vi "Write LEDs.vi"(8 "error in (no error)":errorcluster, 10 "LED Engine Refs in":T1 {"RT IDs"."Slot #" max=15; "RT IDs"."Chip Address (A2 A1 A0)" max=7; "RT Block Data Refs"."Data Reference" format="%.0x"}, 11 "DMA FIFO Ref in":refnum<k20>) -> (0 "error out":errorcluster, 2 "LED Engine Refs out":T1 {"RT IDs"."Slot #" max=15; "RT IDs"."Chip Address (A2 A1 A0)" max=7; "RT Block Data Refs"."Data Reference" format="%.0x"})   [LabVIEW 2014, in "SLSC configuration Engine.lvlib"]
uses:
  SLSC configuration Engine.lvlib
  Type Defs/RT Engine Refs.ctl
  Shared/Type Defs/RT IDs.ctl
  Shared/SPI Utility/Slot #.ctl
  Shared/MCP23S17/Chip Address.ctl
  <vilib>/NI Veristand/Custom Device API/Block Data Reference.ctl
  <vilib>/NI Veristand/Custom Device API/Data Reference.ctl
  <vilib>/NI Veristand/Custom Device API/Global Data Refs.vi
  Shared/Constants.vi
  <vilib>/NI Veristand/Custom Device API/Custom Device API.lvlib
  Shared/SLSC configuration Shared.lvlib
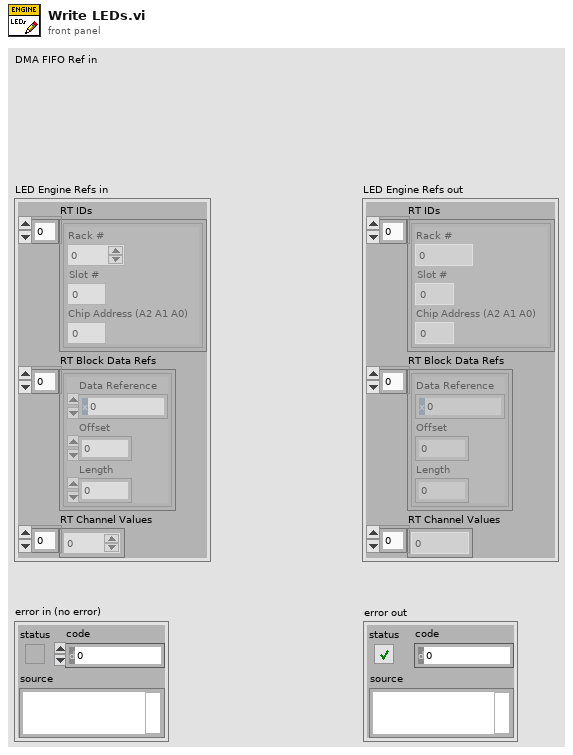
[diagram p1: front panel]
types:
  T1 = typedef "SLSC configuration Engine.lvlib/RT Engine Refs.ctl" = cluster{"RT IDs":T2[], "RT Block Data Refs":T5[], "RT Channel Values":dbl[]}
  T2 = typedef "SLSC configuration Shared.lvlib/RT IDs.ctl" = cluster{"Rack #":u8, "Slot #":T3, "Chip Address (A2 A1 A0)":T4}
  T3 = typedef "SLSC configuration Shared.lvlib/Slot #.ctl" = u8
  T4 = typedef "SLSC configuration Shared.lvlib/Chip Address.ctl" = u8
  T5 = typedef "Custom Device API.lvlib/Block Data Reference.ctl" = cluster{"Data Reference":T6, "Offset":i32, "Length":i32}
  T6 = typedef "Custom Device API.lvlib/Data Reference.ctl" = i32
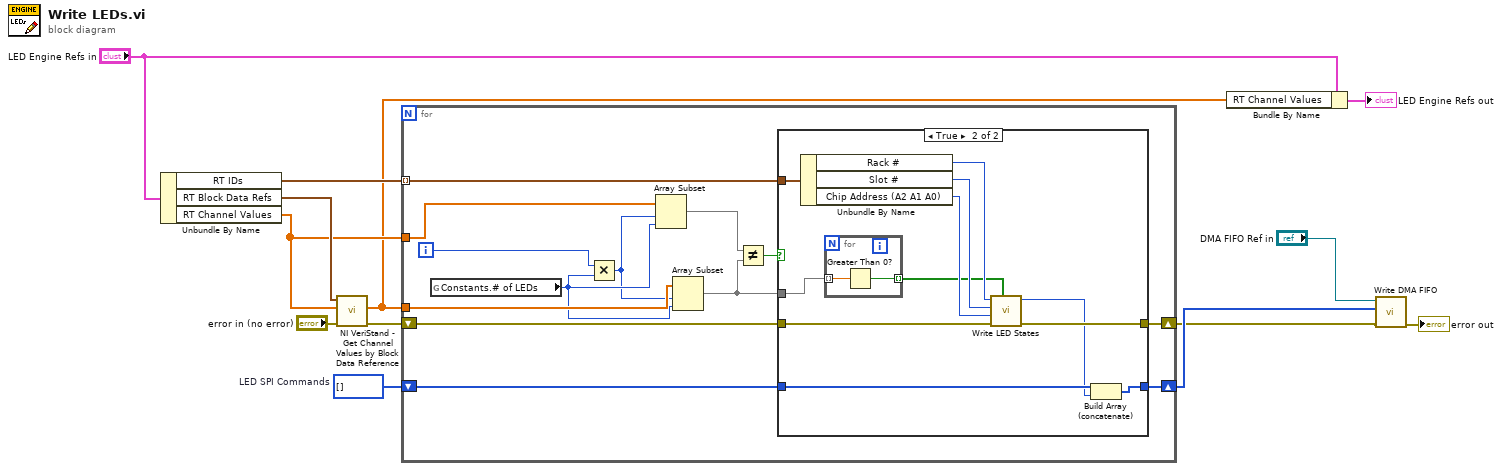
[diagram p0: block diagram]
diagram:
  w5 = u64[] []  # LED SPI Commands
  n1 = Unbundle By Name("LED Engine Refs in") -> ("RT IDs"=w10:T2[], "RT Block Data Refs"=w13:T5[], "RT Channel Values"=w8:dbl[])
  n2 = call <vilib>:"NI VeriStand - Get Channel Values by Block Data Reference.vi"("error in (no error)"="error in (no error)", "Values Array in"=w8, "Block Data Ref"=w13) -> ("error out"=w11:errorcluster, "Values Array out"=w7:dbl[])  [unwired: 6 in, 1 out]
  n3 = for {
    shift-right: [w24] -> w2
    shift-left: w11 -> [w25]
    tunnel: w10 -> [w26] mode=indexing
    tunnel: w7 -> [w17]
    tunnel: w8 -> [w20]
    shift-right: [w21] -> w3
    shift-left: w5 -> [w22]
    i -> [w19]
    n4 = global read "Constants.vi" "Constants.# of LEDs"() -> (w15:u8)
    n5 = Multiply(x=w19, y=w15) -> (x*y=w14:i32)
    n6 = Array Subset(array=w20, index=w14, length=w15) -> (w18:dbl[])
    n7 = Array Subset(array=w17, index=w14, length=w15) -> (w16:dbl[])
    n8 = Not Equal?(x=w18, y=w16) -> (x != y?=w23:bool)
    n9 = case shown="True" w23 {
      tunnel: w26 -> [_ w39]
      tunnel: w25 -> [w28 w38]
      tunnel: w16 -> [_ w30]
      tunnel: [w28 w36] -> w24
      tunnel: w22 -> [w27 w35]
      tunnel: [w27 w33] -> w21
      frame False {
      }
      frame True {
        n10 = Unbundle By Name(w39) -> ("Rack #"=w32:u8, "Slot #"=w31:T3, "Chip Address (A2 A1 A0)"=w37:T4)
        n11 = for {
          tunnel: w30 -> [w41] mode=indexing
          tunnel: [w40] -> w29 mode=indexing
          n12 = Greater Than 0?(x=w41) -> (x > 0?=w40:bool)
        }
        n13 = call "Write LED States.vi"("LED States"=w29, "error in (no error)"=w38, "Chip Address (A2 A1 A0)"=w37, "Slot #"=w31, "Rack #"=w32) -> ("error out"=w36:errorcluster, "FIFO SPI Message"=w34:u64)  [unwired: 4 in, 1 out]
        n14 = Build Array (concatenate)(w35, w34) -> (w33:u64[])
      }
    }
  }
  n15 = Bundle By Name(cluster="LED Engine Refs in", "RT Channel Values"=w7) -> (→"LED Engine Refs out":T1)
  n16 = call "Write DMA FIFO.vi"("error in (no error)"=w2, "FIU SPI Commands"=w3, "DMA FIFO Ref in"="DMA FIFO Ref in") -> ("error out"=→"error out":errorcluster)  [unwired: 8 in]
